vi "Data.Engine.Read Data from HW.vi"(8 "error in":errorcluster, 11 "Data Access API in":refnum<class "Data Access Engine (Express).lvclass">) -> (0 "error out":errorcluster, 3 "Data Access API out":refnum<class "Data Access Engine (Express).lvclass">)   [LabVIEW 2027, in "Data Access Engine (Express).lvlib" / "Data Access Engine (Express).lvclass"]
uses:
  Data Access Engine (Express).lvclass
  Data Access Engine (Express).lvclass/Data Access Engine (Express).ctl
  Access Type Classes/Write/Write.lvclass/Write.ctl
  Access Type Classes/ReadWrite/ReadWrite.lvclass/ReadWrite.ctl
  <userlib>/Custom Device Interfaces_v1.lvlibp/CustomDeviceAPI/Custom Device API.lvclass
  Access Type Classes/ReadWrite/ReadWrite.lvclass
  Access Type Classes/Write/Write.lvclass
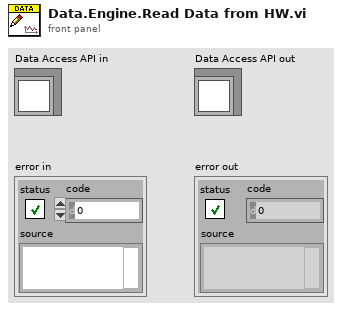
[diagram p1: front panel]
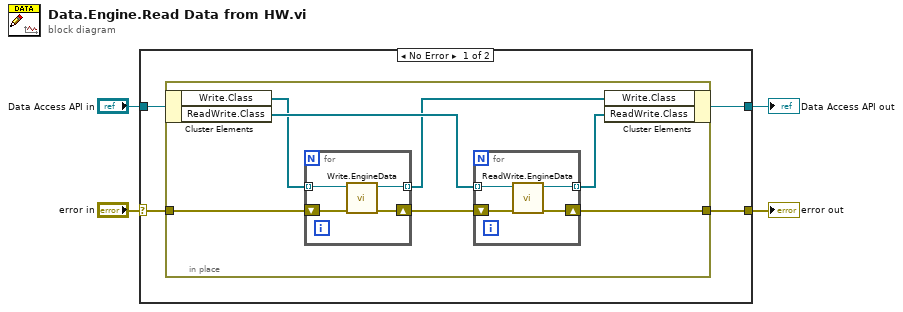
[diagram p0: block diagram]
diagram:
  n1 = case shown="No Error" "error in" {
    selector: "error in" -> [w6 w25]
    tunnel: [w8 w25] -> w3
    tunnel: [w7 w24] -> w1
    tunnel: "Data Access API in" -> [w5 w24]
    frame No Error {
      n2 = in-place {
        in-place-border: w6 -> [w12]
        in-place-border: [w15] -> w8
        n3 = in-place-cluster #1(w5) -> ("Write.Class"=w10:refnum<class "Write.lvclass">[], "ReadWrite.Class"=w14:refnum<class "ReadWrite.lvclass">[])
        n4 = for {
          tunnel: w10 -> [w17] mode=indexing
          shift-right: [w18] -> w11
          shift-left: w12 -> [w19]
          tunnel: [w16] -> w9 mode=indexing
          n5 = call "Write.EngineData.vi"("error in"=w19, "Write in"=w17) -> ("error out"=w18:errorcluster, "Write out"=w16:refnum<class "Write.lvclass">)  [unwired: 8 in]
        }
        n6 = for {
          tunnel: w14 -> [w23] mode=indexing
          shift-right: [w21] -> w15
          shift-left: w11 -> [w22]
          tunnel: [w20] -> w13 mode=indexing
          n7 = call "ReadWrite.EngineData.vi"("error in"=w22, "ReadWrite in"=w23) -> ("error out"=w21:errorcluster, "ReadWrite out"=w20:refnum<class "ReadWrite.lvclass">)  [unwired: 8 in]
        }
        n8 = in-place-cluster #1("Write.Class"=w9, "ReadWrite.Class"=w13) -> (w7:refnum<class "Data Access Engine (Express).lvclass">)
      }
    }
    frame Error {
    }
  }
  "error out" <- w3
  "Data Access API out" <- w1
